vi "ConvertDNetStatuses.vi"(9 "StatusRegister":bool[](array[boolean]), 10 "Status Array":u8[](array[numeric]), 11 "ScanCounter Array":u32[](array[numeric])) -> ()   [LabVIEW 2011]
uses:
  Controls/DNet Status Cluster.ctl
  Controls/DNet StatusRegister Cluster.ctl
  GlobalVariables.vi
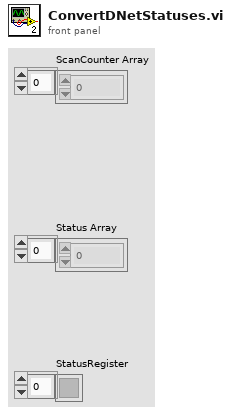
[diagram p1: front panel]
types:
  T1 = typedef "DNet StatusRegister Cluster.ctl" = cluster{"Run":bool, "Fault":bool, "DisableNetwork":bool, "DeviceFailure":bool, "Autoverify":bool, "CommFailure":bool, "DupNodeFail":bool, "DnetPowerDetect":bool}
  T2 = typedef "DNet Status Cluster.ctl" = cluster{"ScanCounter":u32, "DeviceFailureRegister":u8[], "AutoverifyFailureRegister":u8[], "DeviceIdleRegister":u8[], "ActiveNodeRegister":u8[], "StatusDisplay":u8[], "ScannerAddress":u8, "ScannerStatus":u8, "ScrollingDeviceAddress":u8, "ScrollingDeviceStatus":u8}
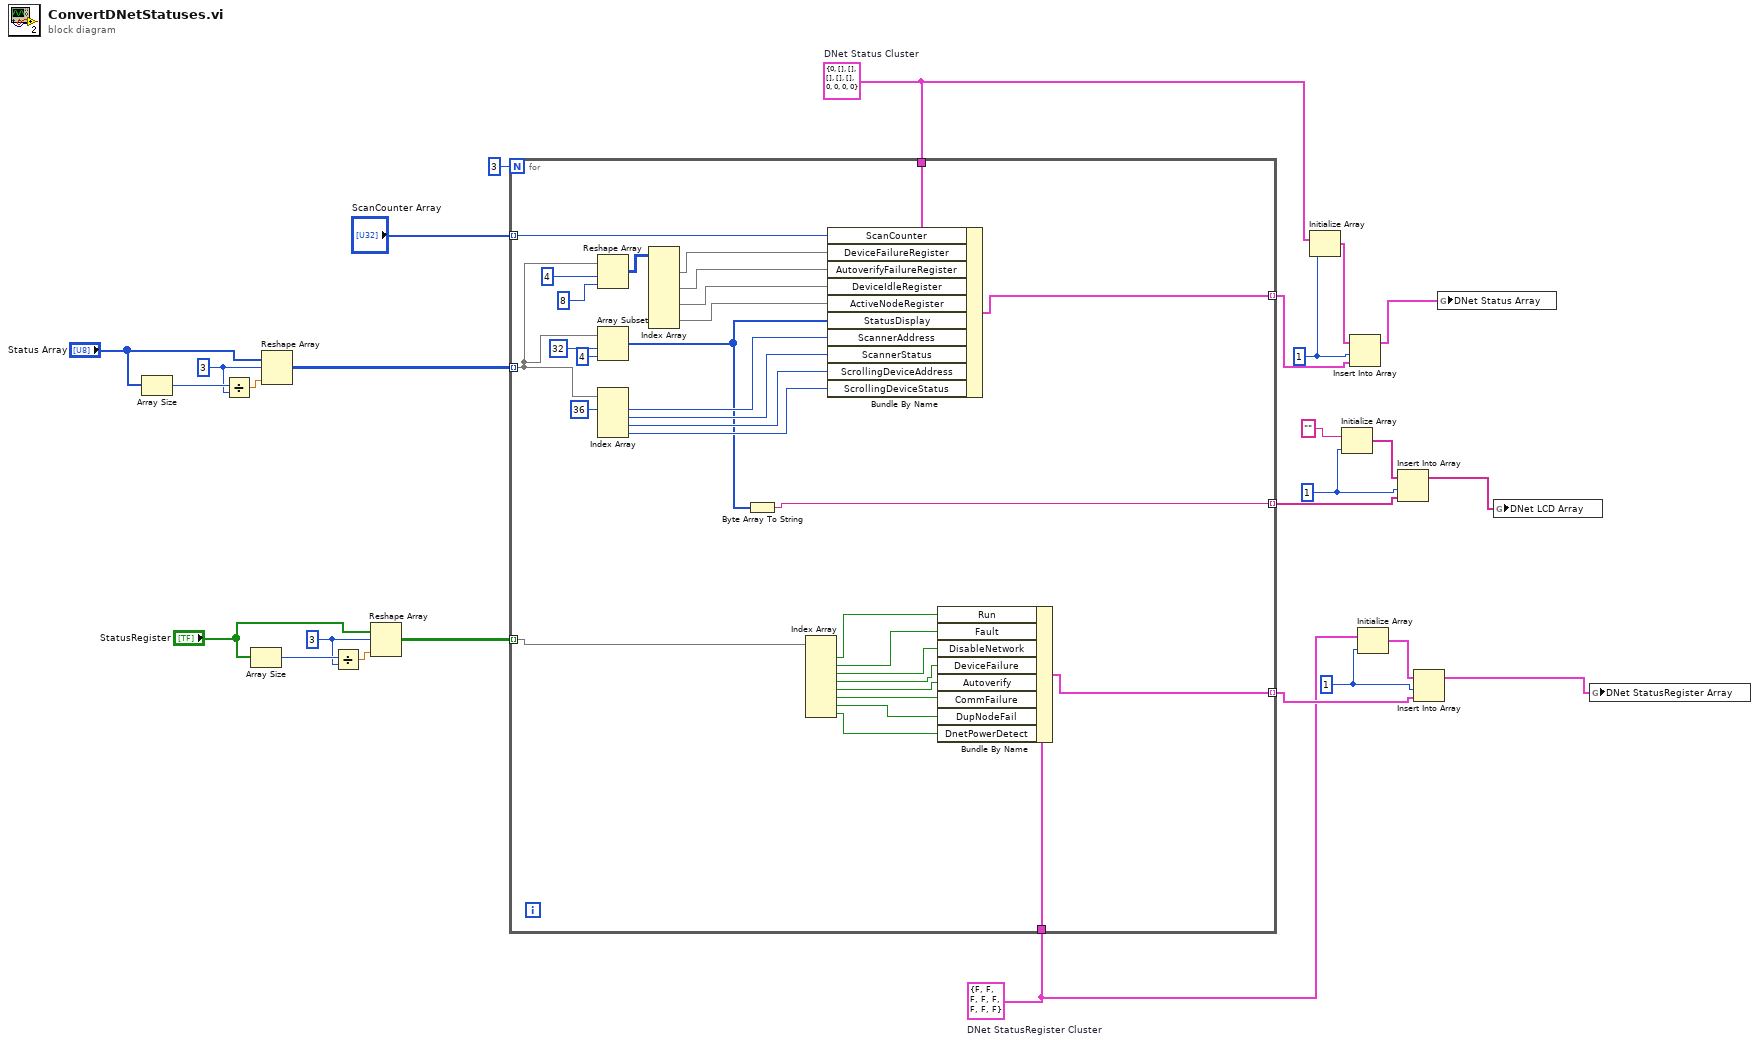
[diagram p0: block diagram]
diagram:
  w4 = T1 {"Run"=FALSE, "Fault"=FALSE, "DisableNetwork"=FALSE, "DeviceFailure"=FALSE, "Autoverify"=FALSE, "CommFailure"=FALSE, "DupNodeFail"=FALSE, "DnetPowerDetect"=FALSE}  # DNet StatusRegister Cluster
  w1 = 1 ("index")
  w2 = 1 ("index")
  w3 = 1 ("index")
  w18 = 3 ("dimension size")
  w22 = 3 ("dimension size")
  w12 = T2 {"ScanCounter"=0, "DeviceFailureRegister"=[], "AutoverifyFailureRegister"=[], "DeviceIdleRegister"=[], "ActiveNodeRegister"=[], "StatusDisplay"=[], "ScannerAddress"=0, "ScannerStatus"=0, "ScrollingDeviceAddress"=0, "ScrollingDeviceStatus"=0}  # DNet Status Cluster
  n1 = Array Size(array="Status Array") -> (size(s)=w24:i32)
  n2 = Divide(x=w24, y=w22) -> (x/y=w23:dbl)
  n3 = Array Size(array="StatusRegister") -> (size(s)=w20:i32)
  n4 = Reshape Array("Status Array", w22, w23) -> (w21:u8[][])
  n5 = Divide(x=w20, y=w18) -> (x/y=w19:dbl)
  n6 = Reshape Array("StatusRegister", w18, w19) -> (w16:bool[][])
  n7 = for {
    N: 3 -> [_]
    tunnel: w12 -> [w58]
    tunnel: "ScanCounter Array" -> [w57] mode=indexing
    tunnel: w21 -> [w34] mode=indexing
    tunnel: w16 -> [w56] mode=indexing
    tunnel: [w47] -> w6 mode=indexing
    tunnel: [w31] -> w15 mode=indexing
    tunnel: [w29] -> w11 mode=indexing
    tunnel: w4 -> [w28]
    n8 = Reshape Array(w34, 4 ("dimension size"), 8 ("dimension size")) -> (w44:u8[][])
    n9 = Array Subset(array=w34, index=32, length=4) -> (w30:u8[])
    n10 = Index Array(array=w34, index #1=36 ("index")) -> (element #1=w36:u8, element #2=w35:u8, element #3=w33:u8, element #4=w32:u8)  [unwired: 3 in]
    n11 = Index Array(array=w44) -> (element #1=w43:u8[], element #2=w42:u8[], element #3=w41:u8[], element #4=w40:u8[])  [unwired: 8 in]
    n12 = Byte Array To String(unsigned byte array=w30) -> (string=w29:string)
    n13 = Index Array(array=w56) -> (element #1=w55:bool, element #2=w54:bool, element #3=w53:bool, element #4=w52:bool, element #5=w51:bool, element #6=w50:bool, element #7=w49:bool, element #8=w48:bool)  [unwired: 8 in]
    n14 = Bundle By Name(cluster=w58, "ScanCounter"=w57, "DeviceFailureRegister"=w43, "AutoverifyFailureRegister"=w42, "DeviceIdleRegister"=w41, "ActiveNodeRegister"=w40, "StatusDisplay"=w30, "ScannerAddress"=w36, "ScannerStatus"=w35, "ScrollingDeviceAddress"=w33, "ScrollingDeviceStatus"=w32) -> (w31:T2)
    n15 = Bundle By Name(cluster=w28, "Run"=w55, "Fault"=w54, "DisableNetwork"=w53, "DeviceFailure"=w52, "Autoverify"=w51, "CommFailure"=w50, "DupNodeFail"=w49, "DnetPowerDetect"=w48) -> (w47:T1)
  }
  n16 = Initialize Array(w12, w3) -> (w13:T2[])
  n17 = Initialize Array("" ("string"), w2) -> (w9:string[])
  n18 = Insert Into Array(array=w13, index=w3, new element=w15) -> (w14:T2[])
  n19 = Initialize Array(w4, w1) -> (w7:T1[])
  n20 = Insert Into Array(array=w9, index=w2, new element=w11) -> (w10:string[])
  n21 = Insert Into Array(array=w7, index=w1, new element=w6) -> (w5:T1[])
  n22 = global write "GlobalVariables.vi" "DNet Status Array"(w14) -> ()
  n23 = global write "GlobalVariables.vi" "DNet LCD Array"(w10) -> ()
  n24 = global write "GlobalVariables.vi" "DNet StatusRegister Array"(w5) -> ()
